vi "10-Tap 8-bit Camera without DRAM (FPGA-SIM)RandomSimDataNoProcessing.vi"() -> ()   [LabVIEW 2013]
doc: "This is the FPGA VI for the 10-Tap 8-Bit Camera with DRAM example. This example demonstrates how to acquire images from a 10-tap, 8-bit, extended configuration, Camera Link camera and transfer the images to the host. This example supports area scan and line scan cameras for both continuous and finite acquisitions.\n\nThis example also demonstrates the use of DRAM as a frame buffer for very high speed acquisitions. Data packing and flow-control are also employed to maximize use of the available DRAM and FIFOs in terms of both memory space and performance.\n\nAdditionally, the example demonstrates the serial server, which allows third-party camera configuration utilities to communicate with the camera using the Camera Link serial interface while this VI is running."
uses:
  Common/CL Signal Mapping.ctl
  Common/CL Configuration.ctl
  FPGA/Sector/Accumulate/Sector Parameter Cluster.ctl
  <vilib>/Platform/TimedLoop/XDataNode/timing_clust.ctl
  <vilib>/Platform/TimedLoop/XDataNode/nitl_modes.ctl
  <vilib>/Platform/TimedLoop/XDataNode/wakeup.ctl
  <vilib>/rvi/Emulation/niFpgaSctlEmulationGetInTimedLoop.vi
  <vilib>/rvi/Emulation/niFpgaEmulationReportErrorSimple.vi
  <vilib>/rvi/Emulation/niFpgaGetClockAttributes.vi
  <vilib>/rvi/Emulation/niFpgaCriticalErrorInLSC.vi
  <vilib>/rvi/FIFO/Fifo_Resource/nirvififoEmulationGetNumberOfElementsToWriteFpgaImpl.vi
  <vilib>/rvi/DataTransferAndStorage/Container/Common/niFpgaContainerGetUniqueNameForEmu.vi
  <vilib>/rvi/FIFO/Fifo_Resource/nirvififoEmulationWriteFpgaImpl.vi
  <vilib>/rvi/FIFO/Fifo_Resource/nirvififoEmulationGetNumberOfElementsToReadFpgaImpl.vi
  <vilib>/rvi/FIFO/Fifo_Resource/nirvififoEmulationReadFpgaImpl.vi
  <vilib>/rvi/Emulation/niFpgaProcessEmulError.vi
  FPGA/Globals/Pixel Location Global.vi
  FPGA/Globals/Sector Parameter Global.vi
  FPGA/Globals/Accumulated Sector Intensity.vi
  <vilib>/Platform/TimedLoop/XDataNode/XDataNode.xnode
  <vilib>/rvi/DataTransferAndStorage/Container/XNode/niFpgaContainer.xnode
  <vilib>/rvi/FIFO/Fifo_Resource/nirvififoEmulationGetNumberOfElementsToWrite.vi
  <vilib>/rvi/FIFO/Fifo_Resource/nirvififoEmulationWrite.vi
  <vilib>/rvi/FIFO/Fifo_Resource/nirvififoEmulationGetNumberOfElementsToRead.vi
  <vilib>/rvi/FIFO/Fifo_Resource/nirvififoEmulationRead.vi
  <vilib>/Platform/TimedLoop/XDataNode/XDNodeRunTimeDep.lvlib
  FPGA/Globals/Wing Square Wave Frequency Global.vi
panel:
  in  "Sim Data":u64=44
  out "Number of Elements to Write Sector Grouping FIFO":u32
  out "Accumulate Ticks":u32
  out "Analysis Ticks":u32
  out "Target Sim TO":bool
  out "Cam Data Timeout":bool
  out "Sector FIFO Timeout":bool
  out "Host DMA Timeout":bool
  out "Number of Elements to Read Cam Data":u32
  out "Number of Elements to Write Host DMA":u32
  in  "Words per image":u32=1000
  in  "Y Resolution":u16=1000
  in  "X Resolution":u16=1000
  in  "[Average BG Intensity]":u8[](array[numeric])=[0, 0, 0, 0, 0, 0, 0, 0, 0, 0, 0, 0, 0, 0, 0, 0, 0, 0, 0, 0, 0, 0, 0, 0, 0, 0, 0, 0, 0, 0, 0, 0]
  in  "Sector Threshold":u8
  in  "# of Frames to Average":u8=1
  in  "Sector Parameters Right":T1={"Start Angle"=0.0, "End Angle"=0.4708251953125, "Inner Radius"=309, "Outter Radius"=405, "Hinge X"=685, "Hinge Y"=527, "NumWingSectors"=8}
  in  "Sector Parameters Left":T1={"Start Angle"=0.65740966796875, "End Angle"=0.99468994140625, "Inner Radius"=309, "Outter Radius"=405, "Hinge X"=464, "Hinge Y"=534, "NumWingSectors"=8}
  in  "CL Config.Configuration":T2=enum."Full"
  in  "CL Config.Signal Mapping":T3=enum."Basler 10-tap"
  in  "CL Config.Line Scan":bool
  in  "CL Config.DVAL Active High":bool=TRUE
  in  "CL Config.LVAL Active High":bool=TRUE
  in  "CL Config.FVAL Active High":bool=TRUE
  in  "CL Config.Spare Active High":bool=TRUE
  in  "Acq Control.Line Scan Height":u32
  in  "Acq Control.Frames To Acq":u32
  in  "Acq Control.Acquire":bool
  in  "Acq Control.Cancel Acq":bool
  in  "Acq Control.Ignore DVAL":bool
  in  "Acq Control.Initialize":bool
  out "Acq Status.Acq In Progress":bool
  out "Acq Status.Clocks Per Line":u32
  out "Acq Status.Frames Acq'd":u32
  out "Acq Status.Lines Per Frame":u32
  out "Acq Status.DMA Write Timeout":bool
  out "Acq Status.Initialized":bool
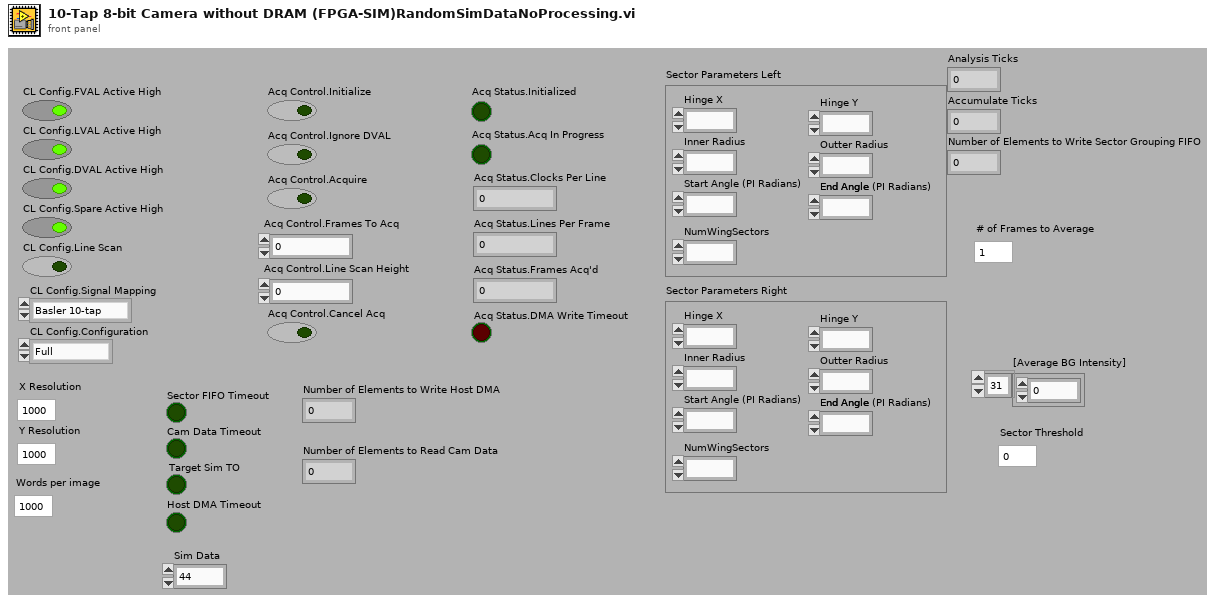
[diagram p1: front panel]
types:
  T1 = typedef "Sector Parameter Cluster.ctl" = cluster{"Start Angle":fxp<+/-,17,2>, "End Angle":fxp<+,17,3>, "Inner Radius":u16, "Outter Radius":u16, "Hinge X":u16, "Hinge Y":u16, "NumWingSectors":u8}
  T2 = typedef "CL Configuration.ctl" = enum8{"Base", "Medium", "Full"}
  T3 = typedef "CL Signal Mapping.ctl" = enum8{"Standard", "Basler 10-tap", "Vosskühler 10-tap"}
  T4 = typedef "XDNodeRunTimeDep.lvlib/timing_clust.ctl" = cluster{"Expected End [f-1]":u64, "Actual End [f-1]":u64, "Finished Late? [f-1]":bool, "Expected End [i-1]":u64, "Actual End [i-1]":u64, "Finished Late? [i-1]":bool, "Expected Start [i]":u64, "Actual Start [i]":u64, "Expected Start [f]":u64, "Actual Start [f]":u64, "Source Name":string, "Structure Name":string, "Period":i64, "Deadline":i64, "Offset":i64, "Start":i64, "Priority":i32, "Timeout":i32, "Mode":T5, "Wakeup Reason":T6, "Error":errorcluster, "Source Type":string, "Secondary Source Type":string, "Global End Time":u64, "Global Start Time":u64, "Frame Duration":u64, "Iteration Duration":u64, "Assigned CPU":i32, "I/O Scan Engine Mode":u32}
  T5 = typedef "XDNodeRunTimeDep.lvlib/nitl_modes.ctl" = enum32{"No Change", "Process missed periods, maintain original phase", "Discard missed periods, maintain original phase", "Process missed periods, ignore original phase", "Discard missed periods, ignore original phase"}
  T6 = typedef "XDNodeRunTimeDep.lvlib/wakeup.ctl" = enum32{"Normal", "Aborted", "Asynchronous wakeup", "Timing source error", "Timed loop error", "Timeout"}
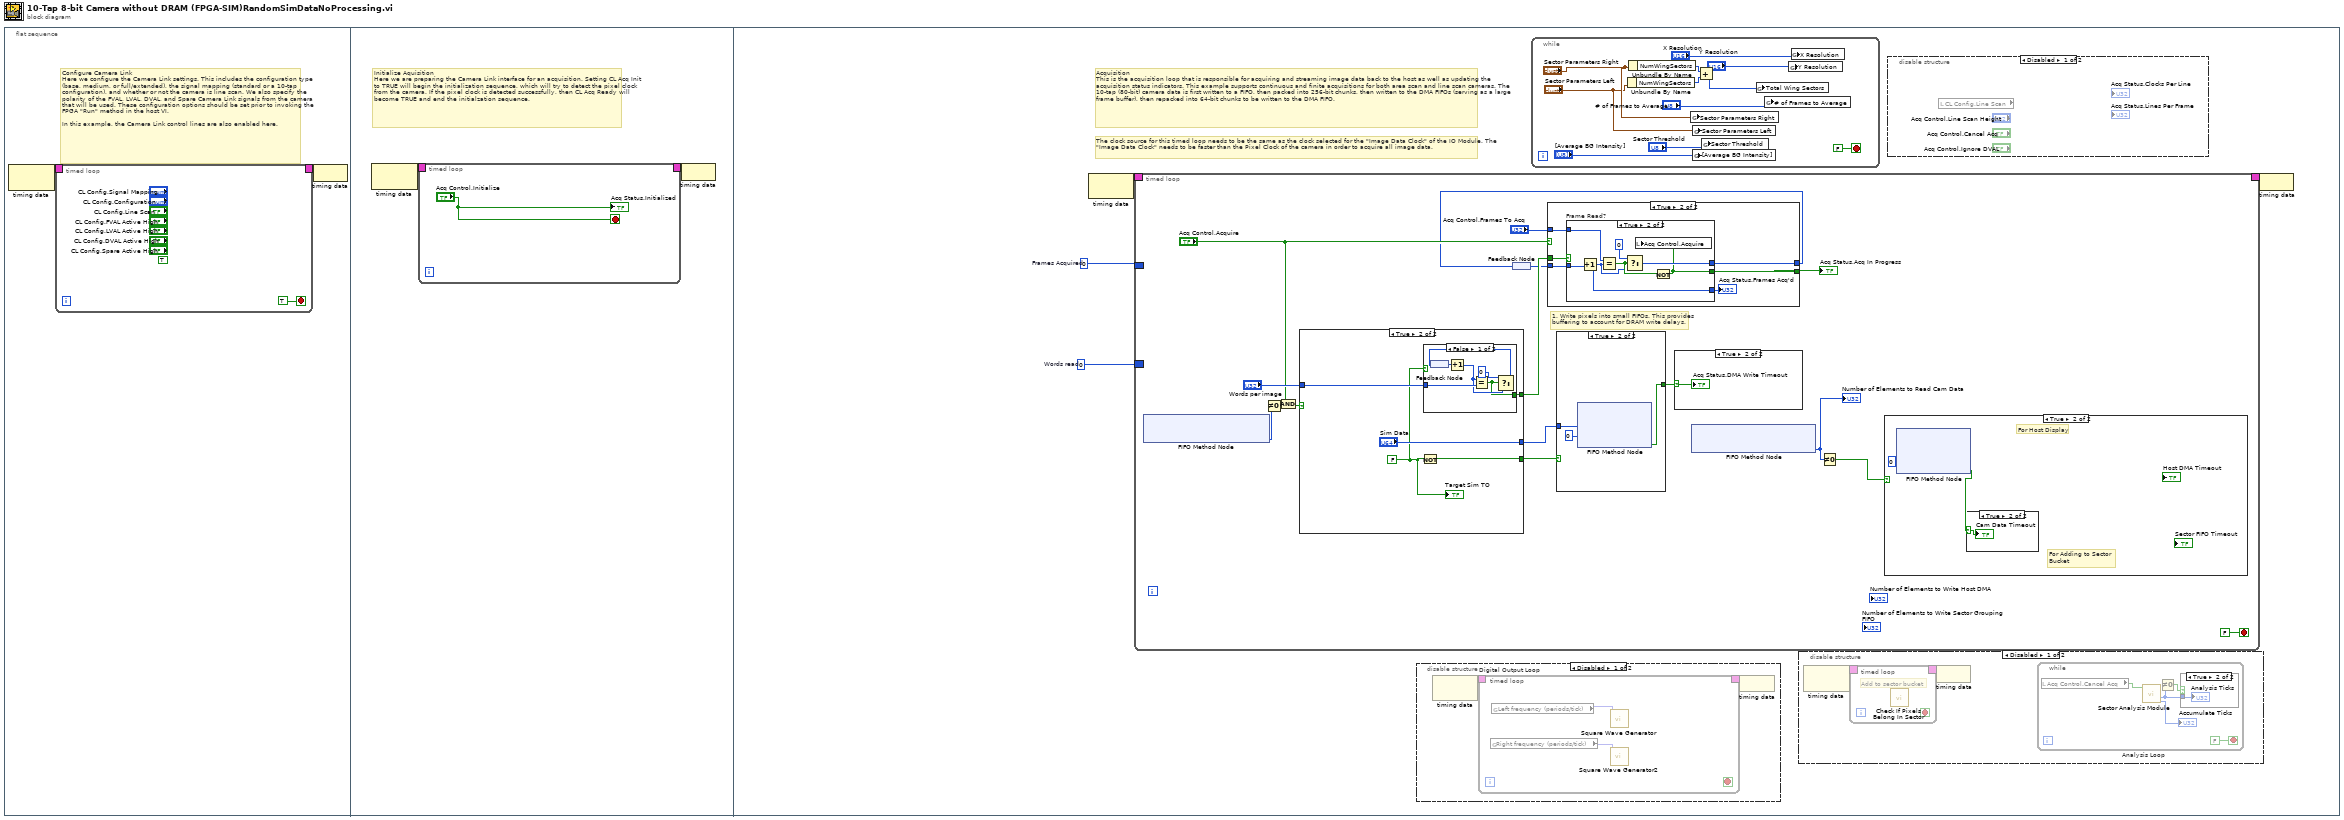
[diagram p0: block diagram]
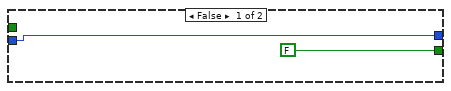
[diagram p7: hidden frame]
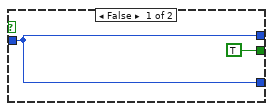
[diagram p8: hidden frame]
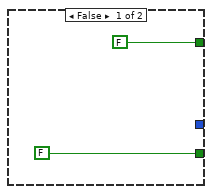
[diagram p9: hidden frame]
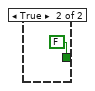
[diagram p10: hidden frame]
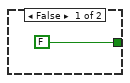
[diagram p13: hidden frame]
diagram:
  n1 = flat-sequence {
    frame #0 {
      # "Configure Camera Link\nHere we configure the Camera Link settings. This includes the configuration type (base, medium, or full/extended), the signal mapping (standard or a 10-tap configuration), and whether or not the camera is line scan. We also specify the polarity of the FVAL, LVAL, DVAL, and Spare Camera Link signals from the camera that will be used. These configuration options should be set prior to invoking the FPGA \"Run\" method in the host VI.\n\nIn this example, the Camera Link control lines are also enabled here."
      n2 = node-c288() -> (w2:T4)  [unwired: 1 in]
      n3 = timed-loop {
        timing: w2 -> [_]
        timing-out: [_] -> w1
        stop <- TRUE stop-if-true
        (unwired) TRUE ("IO Module\\CL Control Enable")
      }
      n4 = node-c288(w1) -> ()
    }
    frame #1 {
      # "Initialize Aquisition\nHere we are preparing the Camera Link interface for an acquisition. Setting CL Acq Init to TRUE will begin the initialization sequence, which will try to detect the pixel clock from the camera. If the pixel clock is detected successfully, then CL Acq Ready will become TRUE and end the initialzation sequence."
      n5 = node-c288() -> (w9:T4)  [unwired: 1 out]
      n6 = timed-loop {
        timing: w9 -> [_]
        timing-out: [_] -> w8
        stop <- "Acq Control.Initialize" stop-if-true
        "Acq Status.Initialized" <- "Acq Control.Initialize"
      }
      n7 = node-c288(w8) -> ()
    }
    frame #2 {
      w15 = u32 0  # Frames Acquired
      w16 = u32 0  # Words read
      # "The clock source for this timed loop needs to be the same as the clock selected for the \"Image Data Clock\" of the IO Module. The \"Image Data Clock\" needs to be faster than the Pixel Clock of the camera in order to acquire all image data."
      # "Acquisition\nThis is the acquisition loop that is responsible for acquiring and streaming image data back to the host as well as updating the acquisition status indicators. This example supports continuous and finite acquisitions for both area scan and line scan cameras. The 10-tap (80-bit) camera data is first written to a FIFO, then packed into 256-bit chunks, then written to the DMA FIFOs (serving as a large frame buffer), then repacked into 64-bit chunks to be written to the DMA FIFO."
      n8 = node-c288() -> (w18:T4)  [unwired: 1 in]
      n9 = timed-loop {
        timing: w18 -> [_]
        timing-out: [_] -> w17
        border: w16 -> [_]
        border: w15 -> [_]
        stop <- FALSE stop-if-true
        # "1. Write pixels into small FIFOs. This provides\nbuffering to account for DRAM write delays."
        n10 = xnode ("FIFO Method Node")() -> ("Number of Elements to Write"=w54:u32)  [unwired: 1 in, 1 out]
        n11 = Not Equal To 0?(x=w54) -> (x != 0?=w53:bool)
        n12 = Compound Arithmetic op=AND("Acq Control.Acquire", w53) -> (w56:bool)
        n13 = case shown="True" w56 {
          tunnel: [_ "Sim Data"] -> w59
          tunnel: [FALSE w82] -> w57
          tunnel: "Words per image" -> [_ w84]
          tunnel: [FALSE w83] -> w50
          frame False {
          }
          frame True {
            w80 = FALSE ("x")
            n14 = Not(x=w80) -> (.not. x?=w82:bool)
            n15 = case shown="False" w80 {
              tunnel: w84 -> [w90 _]
              tunnel: [w85 FALSE] -> w83
              frame False {
                n16 = feedback #1() -> (w89:u32)
                n17 = Increment(x=w89) -> (x+1=w86:u32)
                n18 = Equal?(x=w86, y=w90) -> (x = y?=w85:bool)
                n19 = Select(t=u32 0 ("Acq Status.Frames Acq'd"), s=w85, f=w86) -> (s? t:f=w87:u32)
                n20 = feedback-in #1(w87) -> ()
              }
              frame True {
              }
            }
            "Target Sim TO" <- w80
          }
        }
        n21 = feedback #2() -> (w49:u32)
        n22 = case shown="True" "Acq Control.Acquire" {
          tunnel: w50 -> [_ w68]
          tunnel: w49 -> [w62 w67]
          tunnel: "Acq Control.Frames To Acq" -> [_ w66]
          tunnel: [w62 w65] -> w47
          tunnel: [FALSE w64] -> w46
          frame False {
          }
          frame True {
            n23 = case "Frame Read?" shown="True" w68 {
              tunnel: w67 -> [w69 w77]
              tunnel: w66 -> [_ w76]
              tunnel: [w69 w74] -> w65
              tunnel: [TRUE w72] -> w64
              tunnel: [w69 w71] -> w63
              frame False {
              }
              frame True {
                n24 = Increment(x=w77) -> (x+1=w71:u32)
                n25 = Equal?(x=w76, y=w71) -> (x = y?=w73:bool)
                n26 = Select(t=u32 0 ("Frames Acquired"), s=w73, f=w71) -> (s? t:f=w74:u32)
                n27 = Not(x=w73) -> (.not. x?=w72:bool)
                n28 = local write "Acq Control.Acquire"(w72) -> ()
              }
            }
            "Acq Status.Frames Acq'd" <- w63
          }
        }
        "Acq Status.Acq In Progress" <- w46
        n29 = feedback-in #2(w47) -> ()
        n30 = case shown="True" w57 {
          tunnel: [FALSE ("Timed Out?") w97] -> w45
          tunnel: w59 -> [_ w98]
          frame False {
          }
          frame True {
            n31 = xnode ("FIFO Method Node")("Element"=w98, "Timeout"=0) -> ("Timed Out?"=w97:bool)  [unwired: 1 in, 1 out]
          }
        }
        n32 = case shown="True" w45 {
          selector: w45 -> [_ w60]
          frame False {
          }
          frame True {
            "Acq Status.DMA Write Timeout" <- w60
          }
        }
        n33 = xnode ("FIFO Method Node")() -> ("Number of Elements to Read"=w55:u32)  [unwired: 1 in, 1 out]
        "Number of Elements to Read Cam Data" <- w55
        n34 = Not Equal To 0?(x=w55) -> (x != 0?=w44:bool)
        n35 = case shown="True" w44 {
          frame False {
          }
          frame True {
            # "For Adding to Sector \nBucket"
            # "For Host Display"
            n36 = xnode ("FIFO Method Node")("Timeout"=0) -> ("Timed Out?"=w92:bool)  [unwired: 1 in, 2 out]
            n37 = case shown="True" w92 {
              selector: w92 -> [_ w94]
              frame False {
              }
              frame True {
                "Cam Data Timeout" <- w94
              }
            }
          }
        }
      }
      n38 = disable-structure shown="Disabled" {
        frame Disabled {
          n39 = node-c288() -> (w37:T4)  [unwired: 1 in]
          n40 = timed-loop "Digital Output Loop" {
            timing: w37 -> [_]
            timing-out: [_] -> w36
            stop <- _ stop-if-true
            n41 = global read "Wing Square Wave Frequency Global.vi" "Right frequency (periods/tick)"() -> (w38:fxp<+,32,0>)
            n42 = global read "Wing Square Wave Frequency Global.vi" "Left frequency (periods/tick)"() -> (w39:fxp<+,32,0>)
            n43 = call "Square Wave Generator"("frequency (periods/tick)"=w39) -> ()  [unwired: 14 in, 1 out]
            n44 = call "Square Wave Generator2"("frequency (periods/tick)"=w38) -> ()  [unwired: 14 in, 1 out]
          }
          n45 = node-c288(w36) -> ()
        }
        frame Enabled {
        }
      }
      n46 = while {
        stop <- FALSE stop-if-true
        n47 = Unbundle By Name("Sector Parameters Left") -> ("NumWingSectors"=w111:u8)
        n48 = Unbundle By Name("Sector Parameters Right") -> ("NumWingSectors"=w112:u8)
        n49 = global write "Sector Parameter Global.vi" "Sector Parameters Right"("Sector Parameters Right") -> ()
        n50 = global write "Sector Parameter Global.vi" "Sector Parameters Left"("Sector Parameters Left") -> ()
        n51 = global write "Sector Parameter Global.vi" "[Average BG Intensity]"("[Average BG Intensity]") -> ()
        n52 = Add(x=w112, y=w111) -> (x+y=w110:u8)
        n53 = global write "Sector Parameter Global.vi" "Sector Threshold"("Sector Threshold") -> ()
        n54 = global write "Accumulated Sector Intensity.vi" "Total Wing Sectors"(w110) -> ()
        n55 = global write "Pixel Location Global.vi" "# of Frames to Average"("# of Frames to Average") -> ()
        n56 = global write "Pixel Location Global.vi" "Y Resolution"("Y Resolution") -> ()
        n57 = global write "Pixel Location Global.vi" "X Resolution"("X Resolution") -> ()
      }
      n58 = disable-structure shown="Disabled" {
        frame Disabled {
          n59 = node-c288() -> (w20:T4)  [unwired: 1 in]
          n60 = timed-loop {
            timing: w20 -> [_]
            timing-out: [_] -> w19
            stop <- _ stop-if-true
            # "Add to sector bucket"
            n61 = call "Check If Pixels Belong In Sector.vi"() -> ()  [unwired: 11 in, 1 out]
          }
          n62 = node-c288(w19) -> ()
          n63 = while "Analysis Loop" {
            stop <- FALSE stop-if-true
            n64 = local read "Acq Control.Cancel Acq"() -> (w28:bool)
            n65 = call "Sector Analysis Module.vi"("Canceled?"=w28) -> ("Accumulate Ticks"=→"Accumulate Ticks":u32, "Analysis Ticks"=w26:u32)  [unwired: 8 in, 1 out]
            n66 = Not Equal To 0?(x=w26) -> (x != 0?=w25:bool)
            n67 = case shown="True" w25 {
              tunnel: w26 -> [_ w30]
              frame False {
              }
              frame True {
                "Analysis Ticks" <- w30
              }
            }
          }
        }
        frame Enabled {
        }
      }
      n68 = disable-structure shown="Disabled" {
        frame Disabled {
          n69 = local read "CL Config.Line Scan"() -> (w33:bool)
        }
        frame Enabled {
        }
      }
      n70 = node-c288(w17) -> ()
    }
  }
